vi "Recurse.vi"(6 "Msg Attributes in":refnum<data-value>, 8 "Error in":errorcluster, 11 "TEMPLATE Actor in":refnum<class "TEMPLATE Actor.lvclass">) -> (0 "Error out":errorcluster, 3 "TEMPLATE Actor out":refnum<class "TEMPLATE Actor.lvclass">, 4 "Msg Attributes out":refnum<data-value>)   [LabVIEW 2020, in "_Template.lvlib" / "Templates.lvlib" / "TEMPLATE jettl Actor.lvlib" / "TEMPLATE Actor.lvlib" / "TEMPLATE Actor.lvclass"]
uses:
  TEMPLATE Actor.lvclass
  TEMPLATE Actor.lvclass/TEMPLATE Actor.ctl
  jettl/jettl/jettl.lvlib
  jettl/jettl/Relation.ctl
  jettl/jettl/Teller.ctl
  jettl/jettl/Msg Attributes.ctl
  jettl/jettl/Msg Input/Msg Input.lvclass
  jettl/jettl/Msg Output/Msg Output.lvclass
  jettl/jettl/Msg/Msg.lvclass
  jettl/jettl/Transport/Transport.lvclass
  jettl/jettl/Actor/Actor.lvclass
  jettl/jettl/Msgs.ctl
  jettl/jettl/Unified Layer.ctl
  jettl/jettl/Actor Attributes.ctl
panel:
  # "This front panel should not be manipulated."
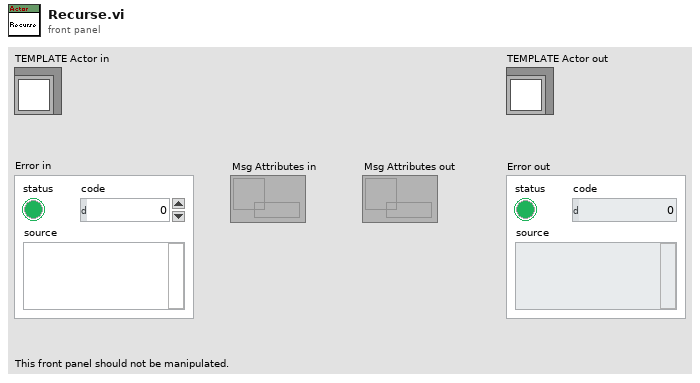
[diagram p1: front panel]
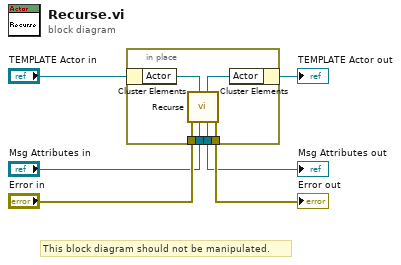
[diagram p0: block diagram]
diagram:
  # "This block diagram should not be manipulated."
  n1 = in-place {
    in-place-border: [w9] -> w6
    in-place-border: "Error in" -> [w10]
    in-place-border: "Msg Attributes in" -> [w7]
    in-place-border: [w8] -> w1
    n2 = in-place-cluster #1("TEMPLATE Actor in") -> ("Actor"=w12:refnum<data-value>)
    n3 = call "Recurse.vi"("Msg Attributes in"=w7, "Actor in"=w12, "Error in"=w10) -> ("Error out"=w9:errorcluster, "Msg Attributes out"=w8:refnum<data-value>, "Actor out"=w11:refnum<data-value>)  [unwired: 6 in]
    n4 = in-place-cluster #1("Actor"=w11) -> (→"TEMPLATE Actor out":refnum<class "TEMPLATE Actor.lvclass">)
  }
  "Error out" <- w6
  "Msg Attributes out" <- w1
